vi "NumericWithScaleFactory.vi"(8 "error in":errorcluster, 11 "Gen Refnum":refnum<vi>) -> (0 "error out":errorcluster, 3 "NumericWithScale out":refnum<class "NumericWithScale.lvclass">)   [LabVIEW 2014, in "NumericWithScale.lvclass"]
uses:
  NumericWithScale.lvclass
  Knob/Knob.lvclass
  Slide/Slide.lvclass
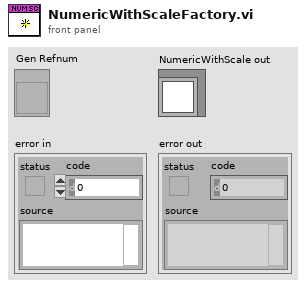
[diagram p1: front panel]
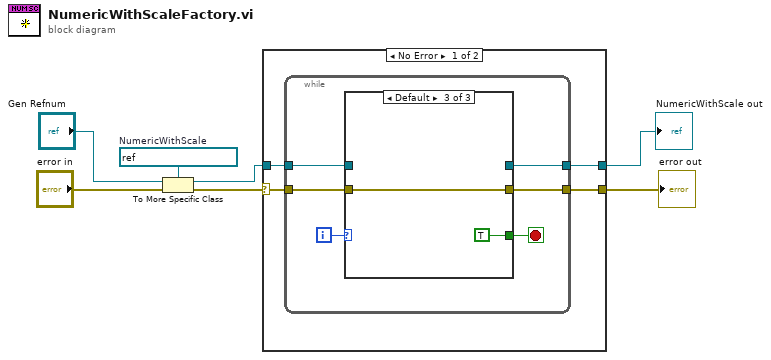
[diagram p0: block diagram]
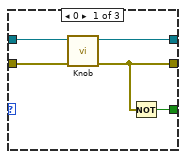
[diagram p2: hidden frame]
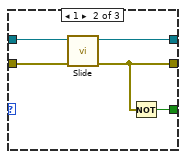
[diagram p3: hidden frame]
diagram:
  w6 = refnum<vi> refnum  # NumericWithScale
  n1 = To More Specific Class(target class=w6, reference="Gen Refnum", error in="error in") -> (specific class reference=w3:refnum<vi>, error out=w4:errorcluster)
  n2 = case shown="No Error" w4 {
    selector: w4 -> [w11 w30]
    tunnel: [w9 _] -> w2
    tunnel: [w8 w30] -> w1
    tunnel: w3 -> [w10 _]
    frame No Error {
      n3 = while {
        tunnel: w11 -> [w16]
        tunnel: [w15] -> w8
        tunnel: [w14] -> w9
        tunnel: w10 -> [w12]
        i -> [w17]
        stop <- w13 stop-if-true
        n4 = case shown="Default" w17 {
          tunnel: w16 -> [w22 w27 w28]
          tunnel: [w19 w24 w28] -> w15
          tunnel: [w21 w26 _] -> w14
          tunnel: [w20 w25 TRUE] -> w13
          tunnel: w12 -> [w18 w23 _]
          frame 0 {
            n5 = call "Knob.vi"("error in"=w22, "Gen Refnum"=w18) -> ("error out"=w19:errorcluster, "Knob out"=w21:refnum<class "Knob.lvclass">)  [unwired: 8 in]
            n6 = Not(x=w19) -> (.not. x?=w20:bool)
          }
          frame 1 {
            n7 = call "Slide.vi"("error in"=w27, "Gen Refnum"=w23) -> ("error out"=w24:errorcluster, "Slide out"=w26:refnum<class "Slide.lvclass">)  [unwired: 8 in]
            n8 = Not(x=w24) -> (.not. x?=w25:bool)
          }
          frame Default {
          }
        }
      }
    }
    frame Error {
    }
  }
  "error out" <- w1
  "NumericWithScale out" <- w2
